vi "Rectangle funct ack completion handler.vi"(11 "Destination folder":path) -> ()   [LabVIEW 2017]
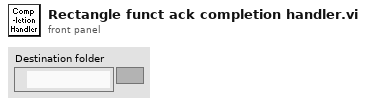
[diagram p1: front panel]
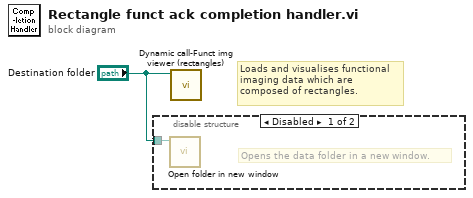
[diagram p0: block diagram]
diagram:
  # "Loads and visualises functional imaging data which are composed of rectangles."
  n1 = disable-structure shown="Disabled" {
    disable-tunnel: "Destination folder" -> [w2 _]
    frame Disabled {
      # "Opens the data folder in a new window."
      n2 = call "Open folder in new window.vi"("Directory to open"=w2) -> ()  [unwired: 10 in, 1 out]
    }
    frame Enabled {
    }
  }
  n3 = call "Dynamic call-Funct img viewer (rectangles).vi"("Experiment Path"="Destination folder") -> ()  [unwired: 10 in, 1 out]
